vi "roboRIO v1.0 Shutdown RSL.vi"(8 "error in (no error)":errorcluster, 10 "Channel List":T3, 11 "myRIO Ref In":T1) -> (0 "error out":errorcluster, 3 "myRIO Ref Out":T1)   [LabVIEW 2021]
uses:
  <vilib>/myRIO/Common/Instrument Driver Framework/roboRIO v1.0/RSL/typedefs/RSL Channels List.ctl
  <vilib>/myRIO/Common/Instrument Driver Framework/roboRIO v1.0/RSL/typedefs/RSL Channels Enum.ctl
  <vilib>/myRIO/Common/Instrument Driver Framework/Utilities/typedefs/myRIO v1.0 Reference.ctl
  <vilib>/myRIO/Common/Instrument Driver Framework/Utilities/typedefs/Generic FPGA Reference.ctl
  <vilib>/myRIO/Common/Instrument Driver Framework/roboRIO v1.0/RSL/typedefs/RSL FPGA Reference.ctl
  <vilib>/Utility/error.llb/Error Cluster From Error Code.vi
  <vilib>/rvi/errors/niLvFpgaAdjustHostInterfaceError.vi
  <vilib>/rvi/interface/nirviReadWriteControl/nirviReadWriteControl.xnode
  <vilib>/rvi/interface/Simulation/niFpgaSimulationCallBeginRW.vi
  NiFpgaLv.dll
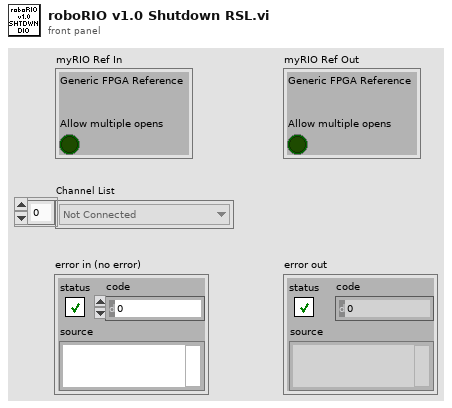
[diagram p1: front panel]
types:
  T1 = typedef "myRIO v1.0 Reference.ctl" = cluster{"Generic FPGA Reference":T2, "Allow multiple opens":bool}
  T2 = typedef "Generic FPGA Reference.ctl" = refnum<k20>
  T3 = typedef "RSL Channels List.ctl" = T4[]
  T4 = typedef "RSL Channels Enum.ctl" = enum16{"Not Connected", "RSL/RSL0"}
  T5 = typedef "RSL FPGA Reference.ctl" = refnum<k20>
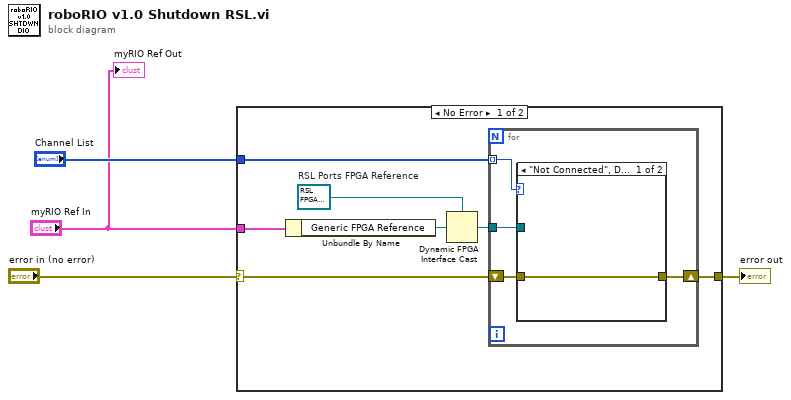
[diagram p0: block diagram]
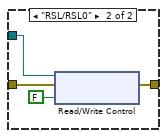
[diagram p2: hidden frame]
diagram:
  n1 = case shown="No Error" "error in (no error)" {
    selector: "error in (no error)" -> [w8 w21]
    tunnel: "myRIO Ref In" -> [w7 _]
    tunnel: [w9 w21] -> w3
    tunnel: "Channel List" -> [w5 _]
    frame No Error {
      w11 = T5 refnum  # RSL Ports FPGA Reference
      n2 = Unbundle By Name(w7) -> ("Generic FPGA Reference"=w6:T2)
      n3 = Dynamic FPGA Interface Cast(Session In=w11, Type=w6) -> (Session Out=w10:T5)
      n4 = for {
        tunnel: w5 -> [w12] mode=indexing
        tunnel: w10 -> [w15]
        shift-right: [w14] -> w9
        shift-left: w8 -> [w13]
        n5 = case shown="\"Not Connected\", Default" w12 {
          tunnel: w15 -> [_ w20]
          tunnel: [w16 w19] -> w14
          tunnel: w13 -> [w16 w18]
          frame "Not Connected", Default {
          }
          frame "RSL/RSL0" {
            n6 = xnode "Read/Write Control"("FPGA VI Reference In"=w20, "error in"=w18, "DO.RSL.OUT"=FALSE) -> ("error out"=w19:errorcluster)  [unwired: 1 out]
          }
        }
      }
    }
    frame Error {
    }
  }
  "error out" <- w3
  "myRIO Ref Out" <- "myRIO Ref In"
